vi "Kinesis - KSG101 - Get Max Travel Range.vi"() -> ()   [LabVIEW 2012]
uses:
  U:/Kinesis LabVIEW Website Examples/Thorlabs.MotionControl.Controls.dll
  Thorlabs.MotionControl.Controls.dll
  U:/Kinesis LabVIEW Website Examples/ThorLabs.MotionControl.KCube.StrainGaugeCLI.dll
  ThorLabs.MotionControl.KCube.StrainGaugeCLI.dll
panel:
  in  "?":bool
  in  "?":bool
  out "Max Travel":dbl
  in  "KCubeStrainGaugeControl":refnum<k24>(container)
  in  "Serial Number":string
  # "Notes:"
  # "- Ensure that the appropriate .DLLs are copied into your Project Folder. Check that the correct bit type are used depending on your version of LabVIEW\ni.e. 32-bit or 64-bit.\n\n\n\n\n\n\n\n\n\n\n\n\n\n\n- Open the example VI through the LabVIEW Project Explorer to correctly load the User Interface from Thorlabs.MotionControl.Controls.dll."
  # "Thorlabs Hardware: KSG101 - K-Cube Strain Gauge Reader\nhttps://www.thorlabs.com/thorproduct.cfm?partnumber=KSG101\n\nDescription: This VI will enable you to connect to the KSG101 Strain Gauge Controller. By clicking the GET MAX TRAVEL button below, you will call GetMaxTravel which gets the maximum travel for the strain gauge, returning the maximum travel for the actuator connected to the strain gauge in 0.1um steps.\n\nInstructions: \n1) Connect your KSG101 device to your PC & power the device, ensuring your stage/actutator is connected. For full device setup, the device product manual can be found on our website here. - https://www.thorlabs.com/thorproduct.cfm?partnumber=KSG101\n2) Enter the device serial number below.\n3) Click 'Run' in the LabVIEW Toolbar.\n4) Click 'GET MAX TRAVEL' after the UI is initialised.\n5) To close the VI, click 'END' below."
  # "Example Image of .NET Controller - VI opened via Project Explorer/ not opened via Project Explorer"
  # "VI Not Opened via Project Explorer"
  # "VI Opened via Project Explorer"
  # "- To explore the range of methods available, please visit the .NET API, included with your Kinesis software.\n\n- For tips on building your own VIs with Thorlabs Motion Control Hardware, please see our LabVIEW Guide here.\nhttps://www.thorlabs.com/newgrouppage9.cfm?objectgroup_id=10285"
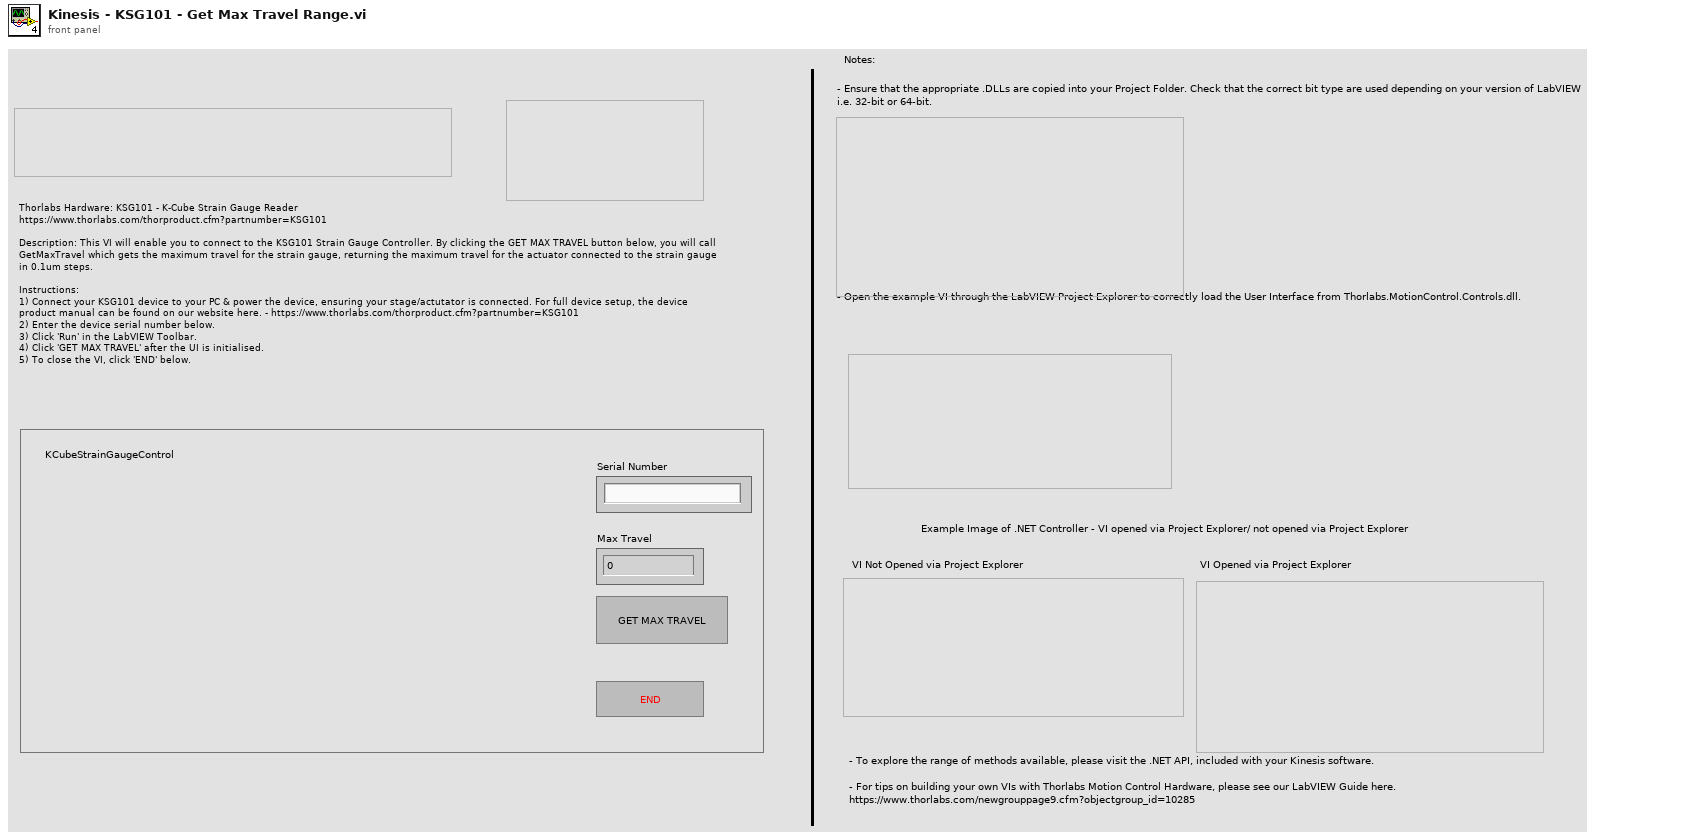
[diagram p1: front panel]
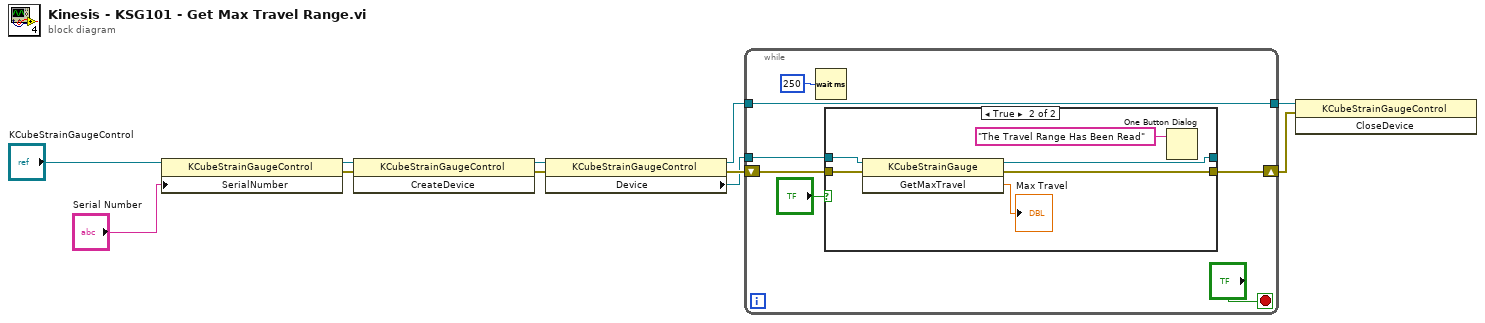
[diagram p0: block diagram]
diagram:
  n1 = property class="KCubeStrainGaugeControl"(reference="KCubeStrainGaugeControl", "SerialNumber"="Serial Number") -> (reference out=w9:refnum<k24>, error out=w7:errorcluster)  [unwired: 1 in]
  n2 = invoke class="KCubeStrainGaugeControl" method="CreateDevice"(reference=w9, error in=w7) -> (reference out=w11:refnum<k24>, error out=w10:errorcluster)  [unwired: 1 in, 1 out]
  n3 = property class="KCubeStrainGaugeControl"(reference=w11, error in=w10) -> (reference out=w4:refnum<k24>, error out=w6:errorcluster, "Device"=w3:refnum<k24>)
  n4 = while {
    shift-right: [w17] -> w1
    shift-left: w6 -> [w18]
    tunnel: w4 -> [w12]
    tunnel: w3 -> [w13]
    tunnel: [w12] -> w2
    stop <- "?" stop-if-true
    n5 = Wait (ms)(milliseconds to wait=u32 250) -> ()  [unwired: 1 out]
    n6 = case shown="True" "?" {
      tunnel: w13 -> [w20 w24]
      tunnel: w18 -> [w19 w23]
      tunnel: [w20 w22] -> _
      tunnel: [w19 w21] -> w17
      frame False {
      }
      frame True {
        n7 = invoke class="KCubeStrainGauge" method="GetMaxTravel"(reference=w24, error in=w23) -> (reference out=w22:refnum<k24>, error out=w21:errorcluster, "GetMaxTravel"=→"Max Travel":dbl)  [unwired: 1 in]
        n8 = One Button Dialog(message="The Travel Range Has Been Read") -> ()  [unwired: 1 in, 1 out]
      }
    }
  }
  n9 = invoke class="KCubeStrainGaugeControl" method="CloseDevice"(reference=w2, error in=w1) -> ()  [unwired: 1 in, 3 out]
